vi "exampleXbox.vi"() -> ()   [LabVIEW 2014]
panel:
  out "Trigger":cluster{"Left":bool, "Right":bool}
  out "Thump":T1
  out "ButtonLed 2":T1
  out "Button3":cluster{"Left":bool, "Right":bool}
  out "Button2":T1
  out "ButtonLed":T1
  in  "stop":bool
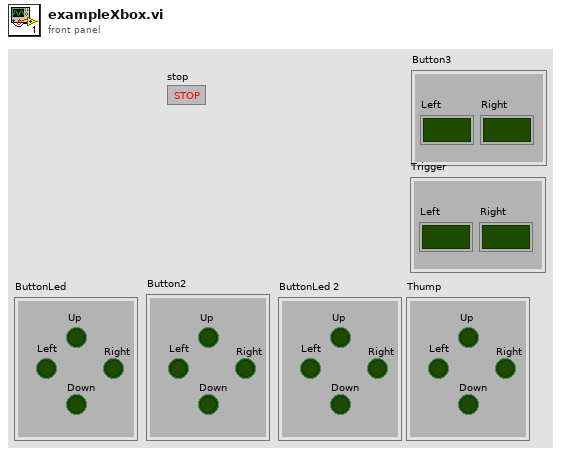
[diagram p1: front panel]
types:
  T1 = cluster{"Down":bool, "Up":bool, "Right":bool, "Left":bool}
  T2 = cluster{"Packet Number":u32, "Gamepad":cluster{"Buttons":u16, "Left Trigger":u8, "Right Trigger":u8, "Thumb LX":i16, "Thumb LY":i16, "Thumb RX":i16, "Thumb RY":i16}}
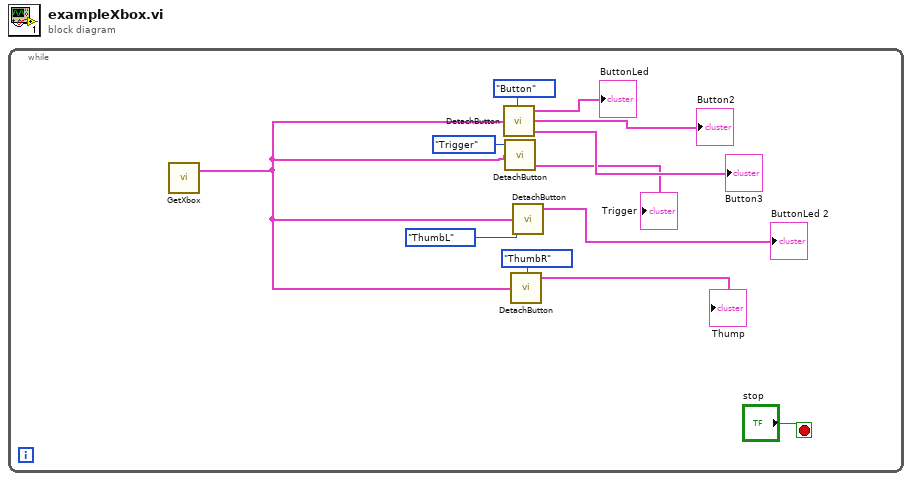
[diagram p0: block diagram]
diagram:
  n1 = while {
    stop <- "stop" stop-if-true
    n2 = call "GetXbox.vi"() -> ("Data Out"=w1:T2)  [unwired: 4 in]
    n3 = call "DetachButton.vi"("pState 2"=w1, "Enum"=enum16{"Button", "ThumbL", "ThumbR", "Trigger"}."Button") -> ("Trigger"=→"Button3":cluster{"Left":bool, "Right":bool}, "Button2"=→"Button2":T1, "Thump"=→"ButtonLed":T1)  [unwired: 1 in]
    n4 = call "DetachButton.vi"("pState 2"=w1, "Enum"=enum16{"Button", "ThumbL", "ThumbR", "Trigger"}."Trigger") -> ("Trigger"=→"Trigger":cluster{"Left":bool, "Right":bool})  [unwired: 1 in, 2 out]
    n5 = call "DetachButton.vi"("pState 2"=w1, "Enum"=enum16{"Button", "ThumbL", "ThumbR", "Trigger"}."ThumbR") -> ("Thump"=→"Thump":T1)  [unwired: 1 in, 2 out]
    n6 = call "DetachButton.vi"("pState 2"=w1, "Enum"=enum16{"Button", "ThumbL", "ThumbR", "Trigger"}."ThumbL") -> ("Thump"=→"ButtonLed 2":T1)  [unwired: 1 in, 2 out]
  }
